vi "imageQ_camera_hook.vi"(6 "timeout in ms (0=don't wait if there are no requests)":i32, 9 "Timestamp/us":u64=2, 10 "ROI":i32[](array[numeric])=[0, 0, 640, 480], 11 "Image":T1) -> ()   [LabVIEW 2019]
uses:
  <vilib>/vision/Image Controls.llb/IMAQ Image.ctl
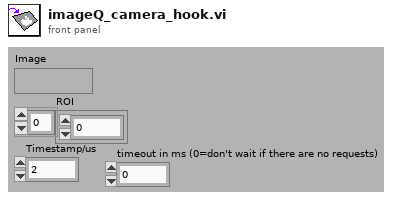
[diagram p1: front panel]
types:
  T1 = typedef "IMAQ Image.ctl" = refnum<image>
  T2 = cluster{"New Image":T1, "queue out":refnum<queue>}
  T3 = cluster{"Image Dst Out":T1, "ROI":i32[], "Timestamp/us":u64}
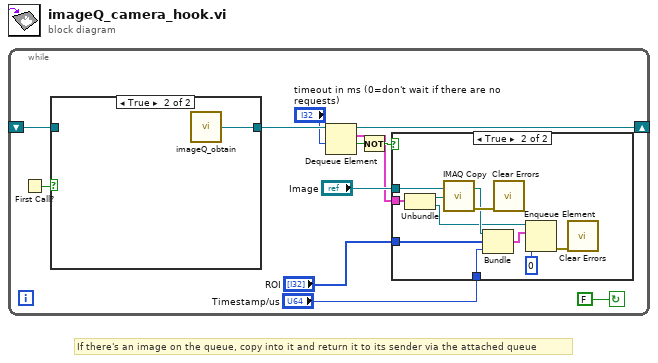
[diagram p0: block diagram]
diagram:
  # "If there's an image on the queue, copy into it and return it to its sender via the attached queue"
  n1 = while {
    shift-right: [w10] -> _
    shift-left: _ -> [w7]
    stop <- FALSE continue-if-true
    n2 = First Call?() -> (First Call?: T/F=w8:bool)
    n3 = case shown="True" w8 {
      tunnel: [w13 w14] -> w12
      tunnel: w7 -> [w13 _]
      frame False {
      }
      frame True {
        n4 = call "imageQ_obtain.vi"() -> ("queue out"=w14:refnum<queue>)
      }
    }
    n5 = Dequeue Element(queue=w12, timeout in ms (-1)="timeout in ms (0=don't wait if there are no requests)") -> (queue out=w10:refnum<queue>, element=w3:T2, timed out?=w9:bool)  [unwired: 1 in, 1 out]
    n6 = Not(x=w9) -> (.not. x?=w5:bool)
    n7 = case shown="True" w5 {
      tunnel: "Image" -> [_ w25]
      tunnel: w3 -> [_ w18]
      tunnel: "ROI" -> [_ w21]
      tunnel: "Timestamp/us" -> [_ w19]
      frame False {
      }
      frame True {
        n8 = Unbundle(w18) -> ("New Image"=w17:T1, "queue out"=w16:refnum<queue>)
        n9 = call "IMAQ Copy"("Image Dst"=w17, "Image Src"=w25) -> ("error out"=w24:errorcluster, "Image Dst Out"=w22:T1)  [unwired: 4 in]
        n10 = Bundle("Image Dst Out"=w22, "ROI"=w21, "Timestamp/us"=w19) -> (w20:T3)  [unwired: 1 in]
        n11 = call <vilib>:"Clear Errors.vi"("error in (no error)"=w24) -> ()  [unwired: 5 in, 2 out]
        n12 = Enqueue Element(queue=w16, element=w20, timeout in ms (-1)=0) -> (error out=w15:errorcluster)  [unwired: 1 in, 2 out]
        n13 = call <vilib>:"Clear Errors.vi"("error in (no error)"=w15) -> ()  [unwired: 5 in, 2 out]
      }
    }
  }
